vi "Actor Core.vi"(8 "error in":errorcluster, 11 "Test in":refnum<class "Test.lvclass">) -> (0 "error out":errorcluster={"status"=TRUE, "code"=1, "source"="Generate User Event in Panel Actor.lvlib:Panel Actor.lvclass:Actor Core.vi:5880003->Test.lvlib:Test.lvclass:Actor Core.vi"}, 3 "Actor out":refnum<class "Actor.lvclass">)   [LabVIEW 2019, in "Test.lvlib" / "Test.lvclass"]
doc: "(<B>Filename</B>: Actor Framework.lvlib:Actor.lvclass:Actor Core.vi)\n\nReceives messages to the actor, reacts to them, and initiates any error handling that may shut the actor down.\n\nDescendant classes may override this VI to append parallel tasks for the actor to complete while it handles messages. Overrides use the Call Parent Method node."
uses:
  Test.lvclass
  C:/Program Files (x86)/National Instruments/LabVIEW 2019/vi.lib/MGI/Panel Manager/Panel Actor/Panel Actor/Panel Actor.lvclass
  <vilib>/ActorFramework/Actor/Actor.lvclass
  <vilib>/ActorFramework/Message Enqueuer/Message Enqueuer.lvclass
  <vilib>/ActorFramework/Message Priority Queue/Message Priority Queue.lvclass
  <vilib>/MGI/Panel Manager/Panel/Panel/Panel.lvclass
  <vilib>/MGI/Panel Manager/Panel/Panel Helper/Panel Helper.lvclass
  <vilib>/MGI/Panel Manager/Panel/Deferer/Deferer.lvclass
  <vilib>/MGI/Panel Manager/Panel/Panel Control Counter/Panel Control Counter.lvclass
  <vilib>/ni/Actors/Network Endpoint Actors/Abstract Classes/Message Stream/Message Stream.lvclass
  Type Defs/Cobra Data.ctl
  Test.lvclass/Test.ctl
  Platform/Platform/Platform.lvclass
  Test Messages/Receive PF Commands Msg/Receive PF Commands Msg.lvclass
  C:/Working Copy/trunk/Modified Cobra Jung/Cobra/Cobra AF/Platform/Platform Messages/Run Msg/PF Commands Msg.lvclass
  Platform/Platform/Platform.lvclass/Platform.ctl
  Instrument/Instrument/Instrument.lvclass
  Power Supply/Power Supply/Power Supply.lvclass
  C:/Working Copy/trunk/Modified Cobra Jung/Cobra/Cobra AF/Instrument/Instrument/Instrument.lvclass
  Test Messages/Receive PS Dataset Msg/Receive PS Dataset Msg.lvclass
  C:/Working Copy/trunk/Modified Cobra Jung/Cobra/Cobra AF/Power Supply/Power Supply Messages/PS Dataset Msg/PS Dataset Msg.lvclass
  Power Supply/Power Supply/Power Supply.lvclass/Power Supply.ctl
  Test Messages/Get Nested Actors Msg/Get Nested Actors Msg.lvclass/Get Nested Actors Msg.ctl
  <vilib>/ActorFramework/Message Enqueuer/Message Enqueuer.lvclass/Message Enqueuer.ctl
  Test Messages/Show Instrument Msg/Show Instrument Msg.lvclass/Show Instrument Msg.ctl
  Test Messages/Update Selected Heads Msg/Update Selected Heads Msg.lvclass/Update Selected Heads Msg.ctl
  Test Messages/Set Cobra Data Msg/Set Cobra Data Msg.lvclass/Set Cobra Data Msg.ctl
  <vilib>/ActorFramework/Message Enqueuer/Enqueue.vi
  <vilib>/MGI/Panel Manager/Panel/Panel/Subpanel/Subpanel.lvclass
  C:/Program Files (x86)/National Instruments/LabVIEW 2019/vi.lib/MGI/Panel Manager/Panel/Panel/Panel.lvclass
  Test Messages/Get Nested Actors Msg/Get Nested Actors Msg.lvclass
  C:/Program Files (x86)/National Instruments/LabVIEW 2019/vi.lib/ActorFramework/Message/Message.lvclass
  Test Messages/Show Instrument Msg/Show Instrument Msg.lvclass
  Test Messages/Update Selected Heads Msg/Update Selected Heads Msg.lvclass
  Test Messages/Set Cobra Data Msg/Set Cobra Data Msg.lvclass
  <vilib>/ActorFramework/Stop Msg/Stop Msg.lvclass
  <vilib>/MGI/Panel Manager/Panel/Panel/Subpanel/Subpanel.vi
  <vilib>/ActorFramework/Message Priority Queue/Priority Enqueue.vi
  <userlib>/_MGI/Application Control/MGI Get Value/MGI Get Value (BOOL).vi
  <vilib>/MGI/Panel Manager/Panel Actor/Panel Actor/Panel Actor.lvclass
  Test.lvlib
  MiniGUI/MiniGUI/LabGUI Head.ctl
  <vilib>/MGI/Panel Manager/Panel/Panel.lvlib
panel:
  out "Run":bool
  out "Connected":bool
  out "IP Address":string
  in  "Test List":i32(listbox)
  in  "Head#2":bool
  in  "Head#1":bool
  out "Data":T1={"M2 Dataset"={"Read Temp"=273.15, "Feedback"=1, "Set Temp"=273.15}, "M1 Dataset"={"Read Temp"=273.15, "Feedback"=1, "Set Temp"=273.15}, "Comp"=FALSE} {"M1 Dataset"."Set Temp" format="%.1f"; "M1 Dataset"."Feedback" items=["Evap Temp", "Case Temp", "Intec Temp", "TSD  Temp", "Autotune", "Extra"]; "M1 Dataset"."Read Temp" format="%.1f"; "M2 Dataset"."Set Temp" format="%.1f"; "M2 Dataset"."Feedback" items=["Evap Temp", "Case Temp", "Intec Temp", "TSD  Temp", "Autotune", "Extra"]; "M2 Dataset"."Read Temp" format="%.1f"}
  # "degC"
  # "degC"
  # "degC"
  # "degC"
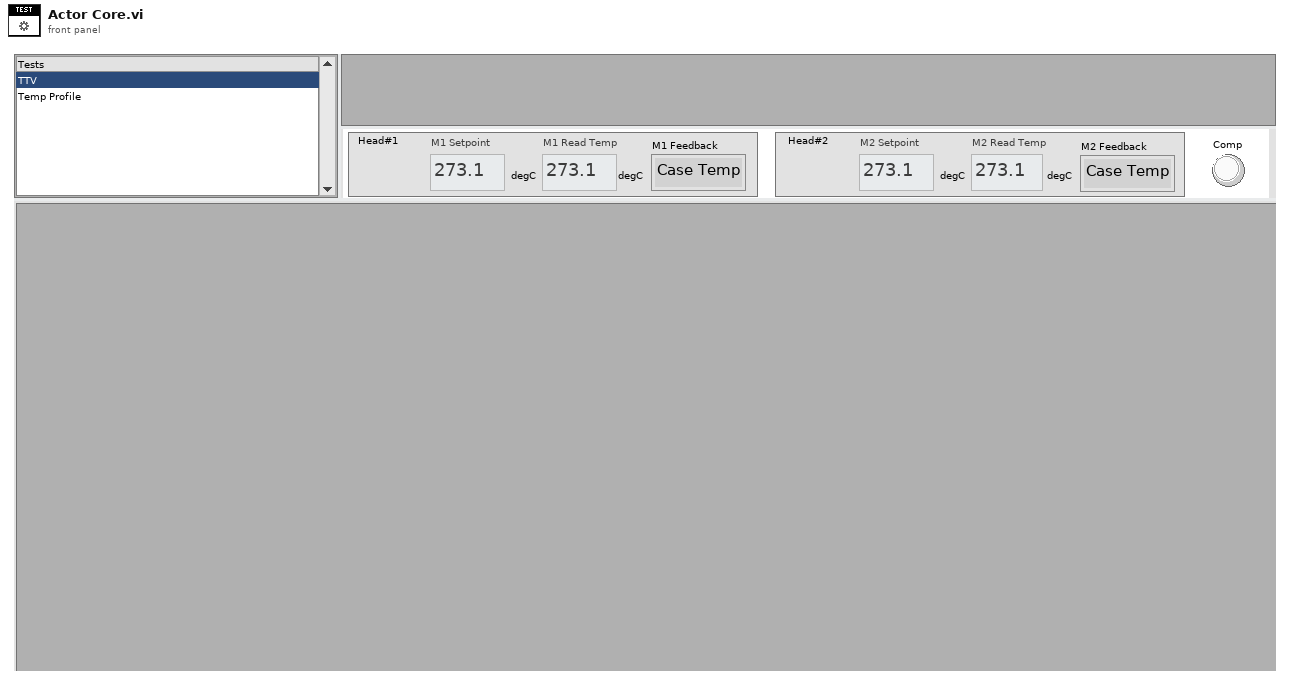
[diagram p1: front panel]
types:
  T1 = typedef "Test.lvlib/Cobra Data.ctl" = cluster{"M2 Dataset":cluster{"Read Temp":dbl, "Feedback":u8, "Set Temp":dbl}, "M1 Dataset":cluster{"Read Temp":dbl, "Feedback":u8, "Set Temp":dbl}, "Comp":bool}
  T2 = enum32{"Invalid", "Standard", "Closed", "Hidden", "Minimized", "Maximized"}
  T3 = cluster{"Event Registration Refnum":refnum<event-registration>, "Pnl Actor":refnum<event-registration>}
  T4 = cluster{"Instrument":refnum<class "Message Enqueuer.lvclass">, "Platform":refnum<class "Message Enqueuer.lvclass">, "Selected Heads":string}
  T5 = typedef "LabGUI Head.ctl" = cluster{"SV":dbl, "PV":dbl, "String":string, "Color Box":u32, "FeedBack":enum16{""}}
  T6 = cluster{"Compressor":bool, "M1":T5, "M2":T5, "Error":string, "System Name":string, "dual head":bool}
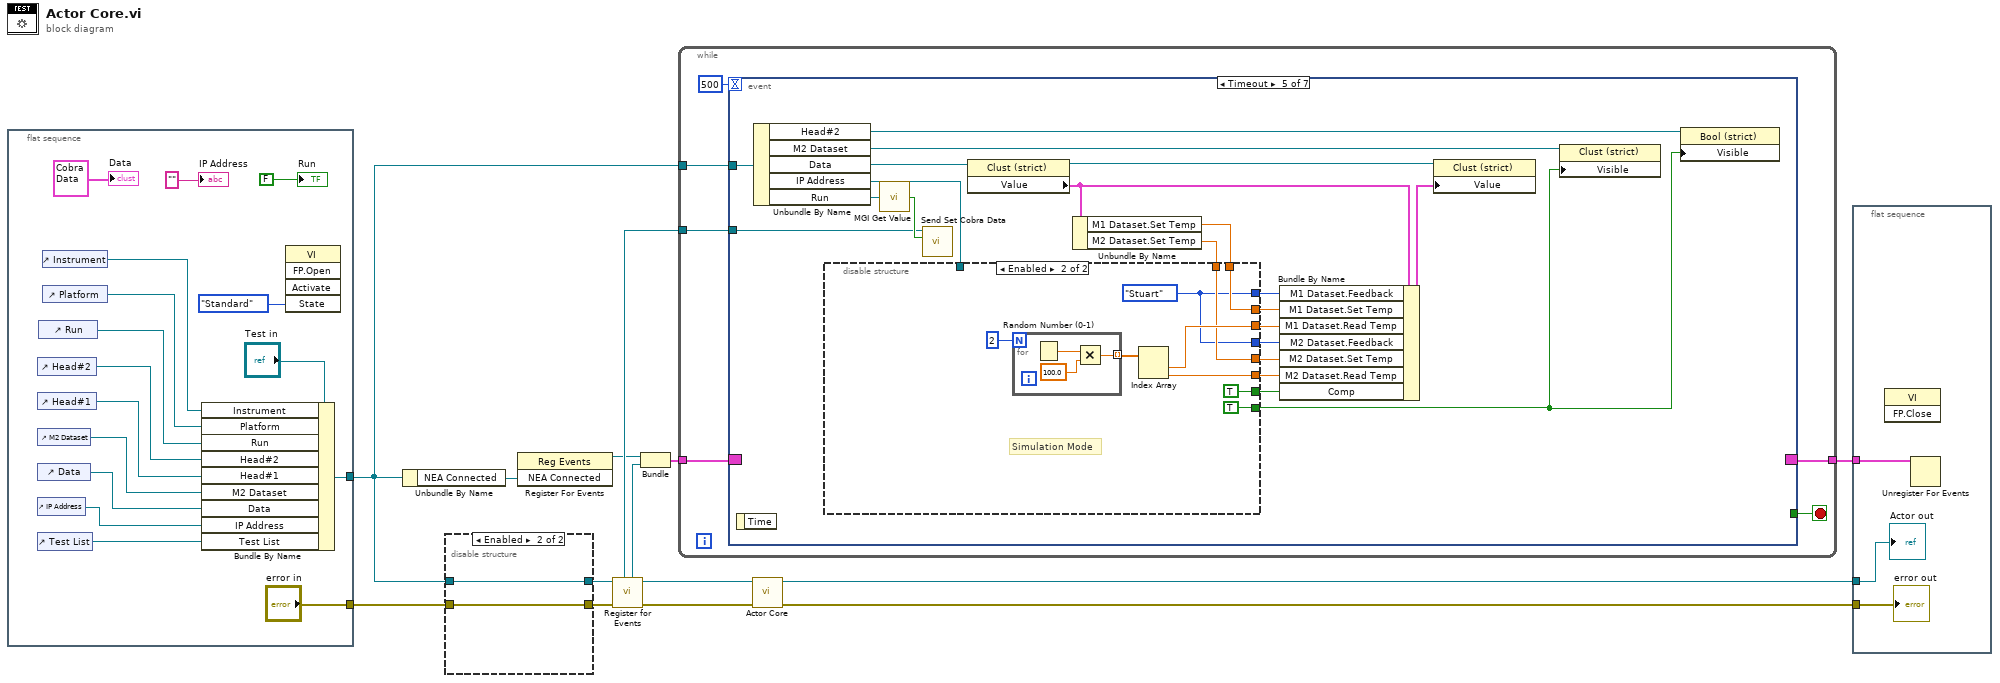
[diagram p0: block diagram]
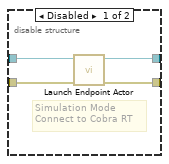
[diagram p2: hidden frame]
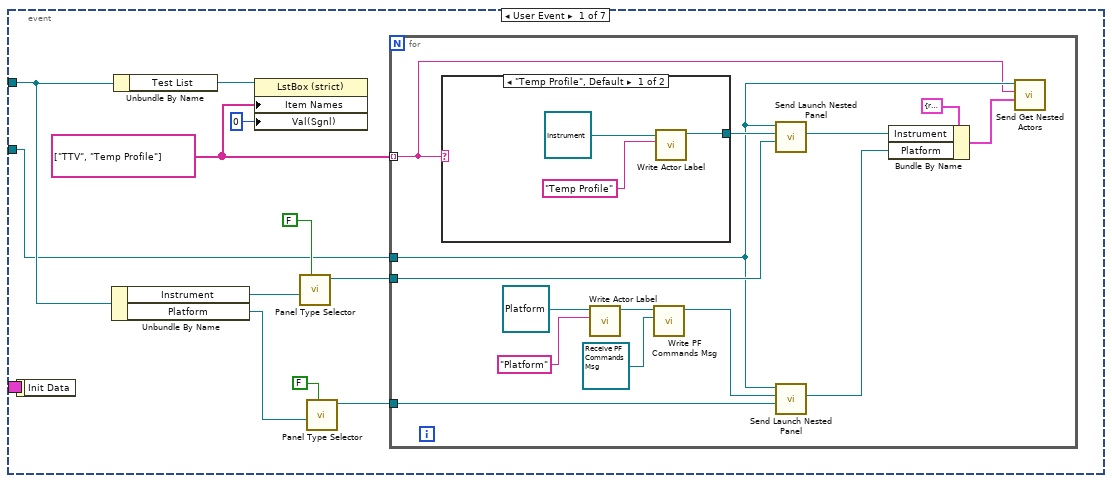
[diagram p3: hidden frame]
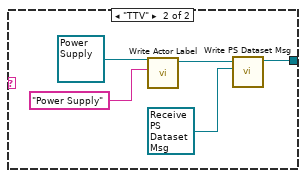
[diagram p4: hidden frame]
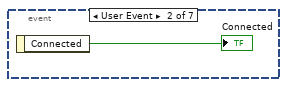
[diagram p5: hidden frame]
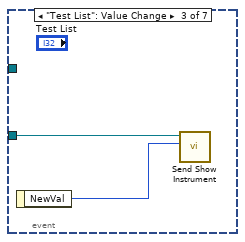
[diagram p6: hidden frame]
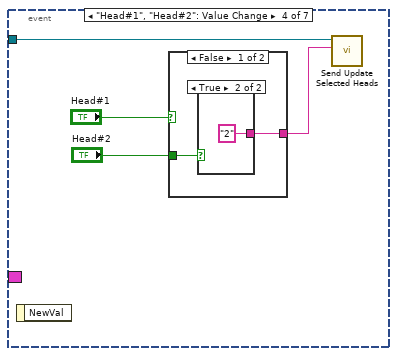
[diagram p7: hidden frame]
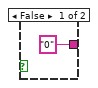
[diagram p8: hidden frame]
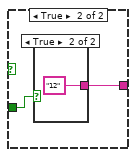
[diagram p9: hidden frame]
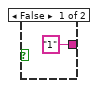
[diagram p10: hidden frame]
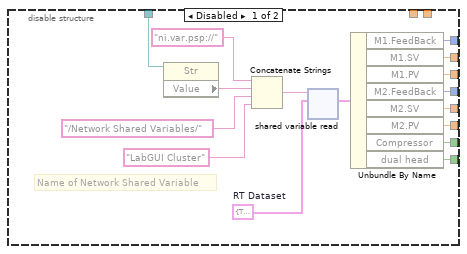
[diagram p11: hidden frame]
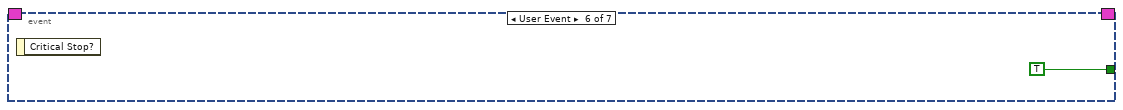
[diagram p12: hidden frame]
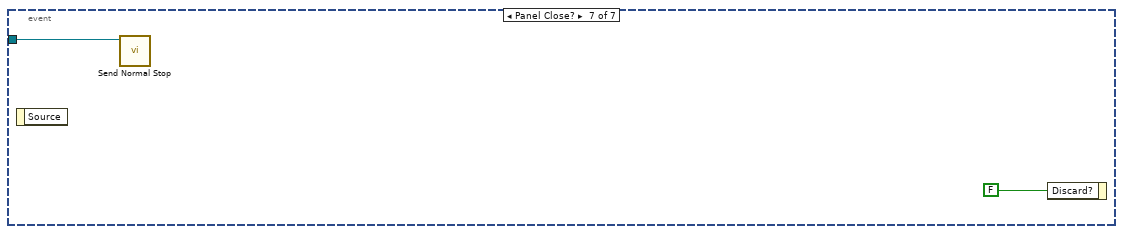
[diagram p13: hidden frame]
diagram:
  n1 = flat-sequence {
    tunnel: [w30] -> w1
    tunnel: ["error in"] -> w2
    frame #0 {
      n2 = control-ref of="Head#2"() -> (w21:refnum<vi>)
      n3 = control-ref of="Head#1"() -> (w22:refnum<vi>)
      n4 = control-ref of="M2 Dataset"() -> (w23:refnum<vi>)
      n5 = control-ref of="Data"() -> (w24:refnum<vi>)
      n6 = control-ref of="IP Address"() -> (w25:refnum<vi>)
      n7 = control-ref of="Test List"() -> (w28:refnum<vi>)
      n8 = control-ref of="Run"() -> (w20:refnum<vi>)
      n9 = control-ref of="Instrument"() -> (w15:refnum<vi>)
      n10 = control-ref of="Platform"() -> (w16:refnum<vi>)
      n11 = Bundle By Name(cluster="Test in", "Instrument"=w15, "Platform"=w16, "Run"=w20, "Head#2"=w21, "Head#1"=w22, "M2 Dataset"=w23, "Data"=w24, "IP Address"=w25, "Test List"=w28) -> (w30:refnum<class "Test.lvclass">)
      n12 = invoke class="VI" method="FP.Open"("State"=T2."Standard") -> ()  [unwired: 4 in, 5 out]
      "IP Address" <- "" ("IP Address")
      "Run" <- FALSE ("Run")
      "Data" <- T1 {"M2 Dataset"={"Read Temp"=273.15, "Feedback"=1, "Set Temp"=273.15}, "M1 Dataset"={"Read Temp"=273.15, "Feedback"=1, "Set Temp"=273.15}, "Comp"=FALSE} ("Data")
    }
  }
  n13 = Unbundle By Name(w1) -> ("NEA Connected"=w6:refnum<user-event>)
  n14 = disable-structure shown="Enabled" {
    disable-tunnel: w2 -> [w34 w35]
    disable-tunnel: [w33 w35] -> w4
    disable-tunnel: w1 -> [w32 w36]
    disable-tunnel: [w31 w36] -> w3
    frame Disabled {
      # "Simulation Mode\nConnect to Cobra RT"
      n15 = call "Launch Endpoint Actor.vi"("error in (no error)"=w34, "Test in"=w32) -> ("error out"=w33:errorcluster, "Test out"=w31:refnum<class "Test.lvclass">)  [unwired: 8 in]
    }
    frame Enabled {
    }
  }
  n16 = register-events(w6) -> (reference out=w5:refnum<event-registration>)  [unwired: 2 in, 1 out]
  n17 = call <vilib>:"Register for Events.vi"("Error In"=w4, "Panel Actor in"=w3) -> ("Error Out"=w13:errorcluster, "Panel Actor out"=w12:refnum<class "Test.lvclass">, "Pnl Actor"=w8:refnum<event-registration>, "Self Enqueuer"=w11:refnum<class "Message Enqueuer.lvclass">)  [unwired: 6 in]
  n18 = Bundle("Event Registration Refnum"=w5, "Pnl Actor"=w8) -> (w7:T3)  [unwired: 1 in]
  n19 = while {
    tunnel: w7 -> [w42]
    tunnel: w11 -> [w41]
    tunnel: [w39] -> w14
    tunnel: w1 -> [w38]
    stop <- w40 stop-if-true
    n20 = event shown="[4] Timeout" {
      selector: w42 -> [_ _ _ _ _ _ _]
      dyn-events: [_ _ _ _ _ _ _] -> w39
      timeout: 500 -> [_ _ _ _ _ _ _]
      tunnel: w41 -> [w43 _ w77 w80 w95 _ w142]
      tunnel: [_ _ _ _ _ TRUE _] -> w40
      tunnel: w38 -> [w44 _ _ _ w111 _ _]
      event User Event {
        w52 = string[] ["TTV", "Temp Profile"]
        n21 = event-data() -> ()  [unwired: 1 in, 1 out]
        n22 = Unbundle By Name(w44) -> ("Instrument"=w47:refnum<vi>, "Platform"=w50:refnum<vi>)
        n23 = Unbundle By Name(w44) -> ("Test List"=w51:refnum<vi>)
        n24 = property class="LstBox (strict)"(reference=w51, "Item Names"=w52, "Val(Sgnl)"=0 ("Value (Signaling)")) -> ()  [unwired: 1 in, 2 out]
        n25 = call-poly <vilib>:"Panel Type Selector.vi"("Autoshow? (T)"=FALSE, "Sub Panel"=w47) -> ("Subpanel Out"=w46:refnum<class "Subpanel.lvclass">)  [unwired: 8 in, 1 out]
        n26 = call-poly <vilib>:"Panel Type Selector.vi"("Autoshow? (T)"=FALSE, "Sub Panel"=w50) -> ("Subpanel Out"=w49:refnum<class "Subpanel.lvclass">)  [unwired: 8 in, 1 out]
        n27 = for {
          tunnel: w46 -> [w62]
          tunnel: w49 -> [w54]
          tunnel: w52 -> [w60] mode=indexing
          tunnel: w43 -> [w61]
          n28 = case shown="\"Temp Profile\", Default" w60 {
            tunnel: [w68 w72] -> w63
            frame "Temp Profile", Default {
              n29 = call-dynamic "Write Actor Label.vi"("Actor Label"="Temp Profile", "Monitored Actor in"=refnum<class "Instrument.lvclass"> refnum ("Instrument.lvlib:Instrument.lvclass")) -> ("Monitored Actor out"=w68:refnum<class "Instrument.lvclass">)  [unwired: 8 in, 1 out]
            }
            frame "TTV" {
              n30 = call-dynamic "Write Actor Label.vi"("Actor Label"="Power Supply", "Monitored Actor in"=refnum<class "Power Supply.lvclass"> refnum ("Power Supply.lvlib:Power Supply.lvclass")) -> ("Monitored Actor out"=w73:refnum<class "Power Supply.lvclass">)  [unwired: 8 in, 1 out]
              n31 = call "Write PS Dataset Msg.vi"("Power Supply.lvlib:PS Dataset Msg.lvclass"=refnum<class "Receive PS Dataset Msg.lvclass"> refnum ("Test.lvlib:Receive PS Dataset Msg.lvclass"), "Power Supply in"=w73) -> ("Power Supply out"=w72:refnum<class "Power Supply.lvclass">)  [unwired: 9 in]
            }
          }
          n32 = call-dynamic "Write Actor Label.vi"("Actor Label"="Platform", "Monitored Actor in"=refnum<class "Platform.lvclass"> refnum ("Platform.lvlib:Platform.lvclass")) -> ("Monitored Actor out"=w67:refnum<class "Platform.lvclass">)  [unwired: 8 in, 1 out]
          n33 = call "Write PF Commands Msg.vi"("Platform.lvlib:PF Commands Msg.lvclass"=refnum<class "Receive PF Commands Msg.lvclass"> refnum ("Test.lvlib:Receive PF Commands Msg.lvclass"), "Platform in"=w67) -> ("Platform out"=w55:refnum<class "Platform.lvclass">)  [unwired: 9 in]
          n34 = call <vilib>:"Send Launch Nested Panel.vi"("Panel"=w62, "Nested Panel Actor"=w63, "Self Enqueuer in"=w61) -> ("Nested Actor's Enqueuer"=w58:refnum<class "Message Enqueuer.lvclass">)  [unwired: 7 in, 1 out]
          n35 = call <vilib>:"Send Launch Nested Panel.vi"("Panel"=w54, "Nested Panel Actor"=w55, "Self Enqueuer in"=w61) -> ("Nested Actor's Enqueuer"=w57:refnum<class "Message Enqueuer.lvclass">)  [unwired: 7 in, 1 out]
          n36 = Bundle By Name(cluster=T4 {"Instrument"=refnum, "Platform"=refnum, "Selected Heads"="0"} ("Nested Actors"), "Instrument"=w58, "Platform"=w57) -> (w56:T4)
          n37 = call "Send Get Nested Actors.vi"("Nested Actors"=w56, "key"=w60, "Message Enqueuer"=w61) -> ()  [unwired: 7 in, 2 out]
        }
      }
      event User Event {
        n38 = event-data() -> ("Connected"=→"Connected":bool)  [unwired: 1 in]
      }
      event "Test List": Value Change {
        n39 = event-data() -> ("NewVal"=w78:i32)  [unwired: 1 in]
        n40 = call "Send Show Instrument.vi"("Test"=w78, "Message Enqueuer"=w77) -> ()  [unwired: 8 in, 2 out]
      }
      event "Head#1", "Head#2": Value Change {
        n41 = event-data() -> ()  [unwired: 1 in, 1 out]
        n42 = case shown="False" "Head#1" {
          tunnel: "Head#2" -> [w84 w88]
          tunnel: [w83 w87] -> w79
          frame False {
            n43 = case shown="True" w84 {
              tunnel: ["0" ("Value") "2" ("Value")] -> w83
              frame False {
              }
              frame True {
              }
            }
          }
          frame True {
            n44 = case shown="True" w88 {
              tunnel: ["1" ("Value") "12" ("Value")] -> w87
              frame False {
              }
              frame True {
              }
            }
          }
        }
        n45 = call "Send Update Selected Heads.vi"("Selected Heads"=w79, "Message Enqueuer"=w80) -> ()  [unwired: 8 in, 2 out]
      }
      event Timeout {
        n46 = event-data() -> ()  [unwired: 1 in, 1 out]
        n47 = Unbundle By Name(w111) -> ("Head#2"=w102:refnum<vi>, "M2 Dataset"=w100:refnum<vi>, "Data"=w98:refnum<vi>, "IP Address"=w110:refnum<vi>, "Run"=w94:refnum<vi>)
        n48 = call-poly <userlib>:"MGI Get Value.vi"("Ref"=w94) -> ("Value"=w96:bool)
        n49 = call "Send Set Cobra Data.vi"("Run"=w96, "Message Enqueuer"=w95) -> ()  [unwired: 8 in, 2 out]
        n50 = property class="Clust (strict)"(reference=w98) -> (reference out=w99:refnum<vi>, "Value"=w93:T1)  [unwired: 1 in, 1 out]
        n51 = Unbundle By Name(w93) -> ("M1 Dataset.Set Temp"=w92:dbl, "M2 Dataset.Set Temp"=w91:dbl)
        n52 = disable-structure shown="Enabled" {
          disable-tunnel: w110 -> [w127 _]
          disable-tunnel: [w125 w128] -> w109
          disable-tunnel: [w124 w130] -> w108
          disable-tunnel: [w123 w132] -> w107
          disable-tunnel: [w122 w128] -> w106
          disable-tunnel: [w121 w129] -> w105
          disable-tunnel: [w120 w131] -> w104
          disable-tunnel: [w119 TRUE ("Compressor")] -> w103
          disable-tunnel: [w118 TRUE ("dual head")] -> w101
          disable-tunnel: w92 -> [_ w130]
          disable-tunnel: w91 -> [_ w129]
          frame Disabled {
            w112 = T6 {"Compressor"=TRUE, "M1"={"SV"=100.0, "PV"=200.0, "String"="", "Color Box"=6618880, "FeedBack"=enum.""}, "M2"={"SV"=300.0, "PV"=400.0, "String"="", "Color Box"=16725248, "FeedBack"=enum.""}, "Error"="", "System Name"="", "dual head"=TRUE}  # RT Dataset
            # "Name of Network Shared Variable"
            n53 = property class="Str"(reference=w127) -> ("Value"=w113:string)  [unwired: 1 in, 2 out]
            n54 = Concatenate Strings("ni.var.psp://", w113, "/Network Shared Variables/", "LabGUI Cluster") -> (w115:string)
            n55 = shared-variable-read(w115, w112) -> (w126:T6)  [unwired: 1 in, 3 out]
            n56 = Unbundle By Name(w126) -> ("M1.FeedBack"=w125:enum16{""}, "M1.SV"=w124:dbl, "M1.PV"=w123:dbl, "M2.FeedBack"=w122:enum16{""}, "M2.SV"=w121:dbl, "M2.PV"=w120:dbl, "Compressor"=w119:bool, "dual head"=w118:bool)
          }
          frame Enabled {
            w128 = enum16{"Stuart"}."Stuart" ("FeedBack")
            # "Simulation Mode"
            n57 = for {
              N: 2 -> [_]
              tunnel: [w137] -> w134 mode=indexing
              n58 = Random Number (0-1)() -> (number: 0 to 1=w138:dbl)
              n59 = Multiply(x=w138, y=100.0) -> (x*y=w137:dbl)
            }
            n60 = Index Array(array=w134) -> (element #1=w132:dbl, element #2=w131:dbl)  [unwired: 2 in]
          }
        }
        n61 = Bundle By Name(cluster=w93, "M1 Dataset.Feedback"=w109, "M1 Dataset.Set Temp"=w108, "M1 Dataset.Read Temp"=w107, "M2 Dataset.Feedback"=w106, "M2 Dataset.Set Temp"=w105, "M2 Dataset.Read Temp"=w104, "Comp"=w103) -> (w97:T1)
        n62 = property class="Clust (strict)"(reference=w99, "Value"=w97) -> ()  [unwired: 1 in, 2 out]
        n63 = property class="Clust (strict)"(reference=w100, "Visible"=w101) -> ()  [unwired: 1 in, 2 out]
        n64 = property class="Bool (strict)"(reference=w102, "Visible"=w101) -> ()  [unwired: 1 in, 2 out]
      }
      event User Event {
        n65 = event-data() -> ()  [unwired: 1 in, 1 out]
      }
      event Panel Close? {
        n66 = event-data() -> ()  [unwired: 1 in, 1 out]
        n67 = call <vilib>:"Send Normal Stop.vi"("Message Enqueuer"=w142) -> ()  [unwired: 10 in, 1 out]
        n68 = event-data("Discard?"=FALSE) -> ()  [unwired: 1 in, 1 out]
      }
    }
  }
  n69 = call-parent "Actor Core.vi"("error in"=w13, "Panel Actor in"=w12) -> ("error out"=w10:errorcluster, "Actor out"=w9:refnum<class "Actor.lvclass">)  [unwired: 8 in]
  n70 = flat-sequence {
    tunnel: w14 -> [w145]
    tunnel: w10 -> [w143]
    tunnel: w9 -> [w144]
    frame #0 {
      n71 = invoke class="VI" method="FP.Close"() -> ()  [unwired: 3 in, 3 out]
      n72 = Unregister For Events(event registration refnum=w145) -> ()  [unwired: 1 in, 1 out]
      "error out" <- w143
      "Actor out" <- w144
    }
  }
